vi "PathVelocityProfile.vi"(0 "Pose":dbl[](array[numeric]), 1 "time":dbl, 3 "intervalo":dbl=0.016, 5 "estimatives":T2, 9 "Path  Smooth":dbl[][](array[numeric]), 11 "V_max":dbl format="%#_13g", 13 "Accel":dbl=10.0, 14 "DesAccel":dbl=15.0) -> (4 "Time X":dbl[](array[numeric]), 6 "Velocities X":dbl[](array[numeric]), 8 "Time Y":dbl[](array[numeric]), 10 "Velocities Y":dbl[](array[numeric]))   [LabVIEW 2017]
uses:
  Controle/VelocityProfileState.ctl
  <vilib>/Analysis/_algsub.llb/Real Vector Norm.vi
  <vilib>/Analysis/coordinate.llb/Wrap Angle (scalar).vi
  <vilib>/Analysis/NI_AAL_Angle.lvlib
  <vilib>/Analysis/NI_AALPro.lvlib
panel:
  in  "est_vy":dbl
  in  "est_vx":dbl
  out "VelocityProfile Y":T1[](array[typedef])
  out "VelocityProfile X":T1[](array[typedef])
  out "Velocity Profile Y":cluster{dbl[], dbl[]}[](graph)
  out "Velocity Profile X":cluster{dbl[], dbl[]}[](graph)
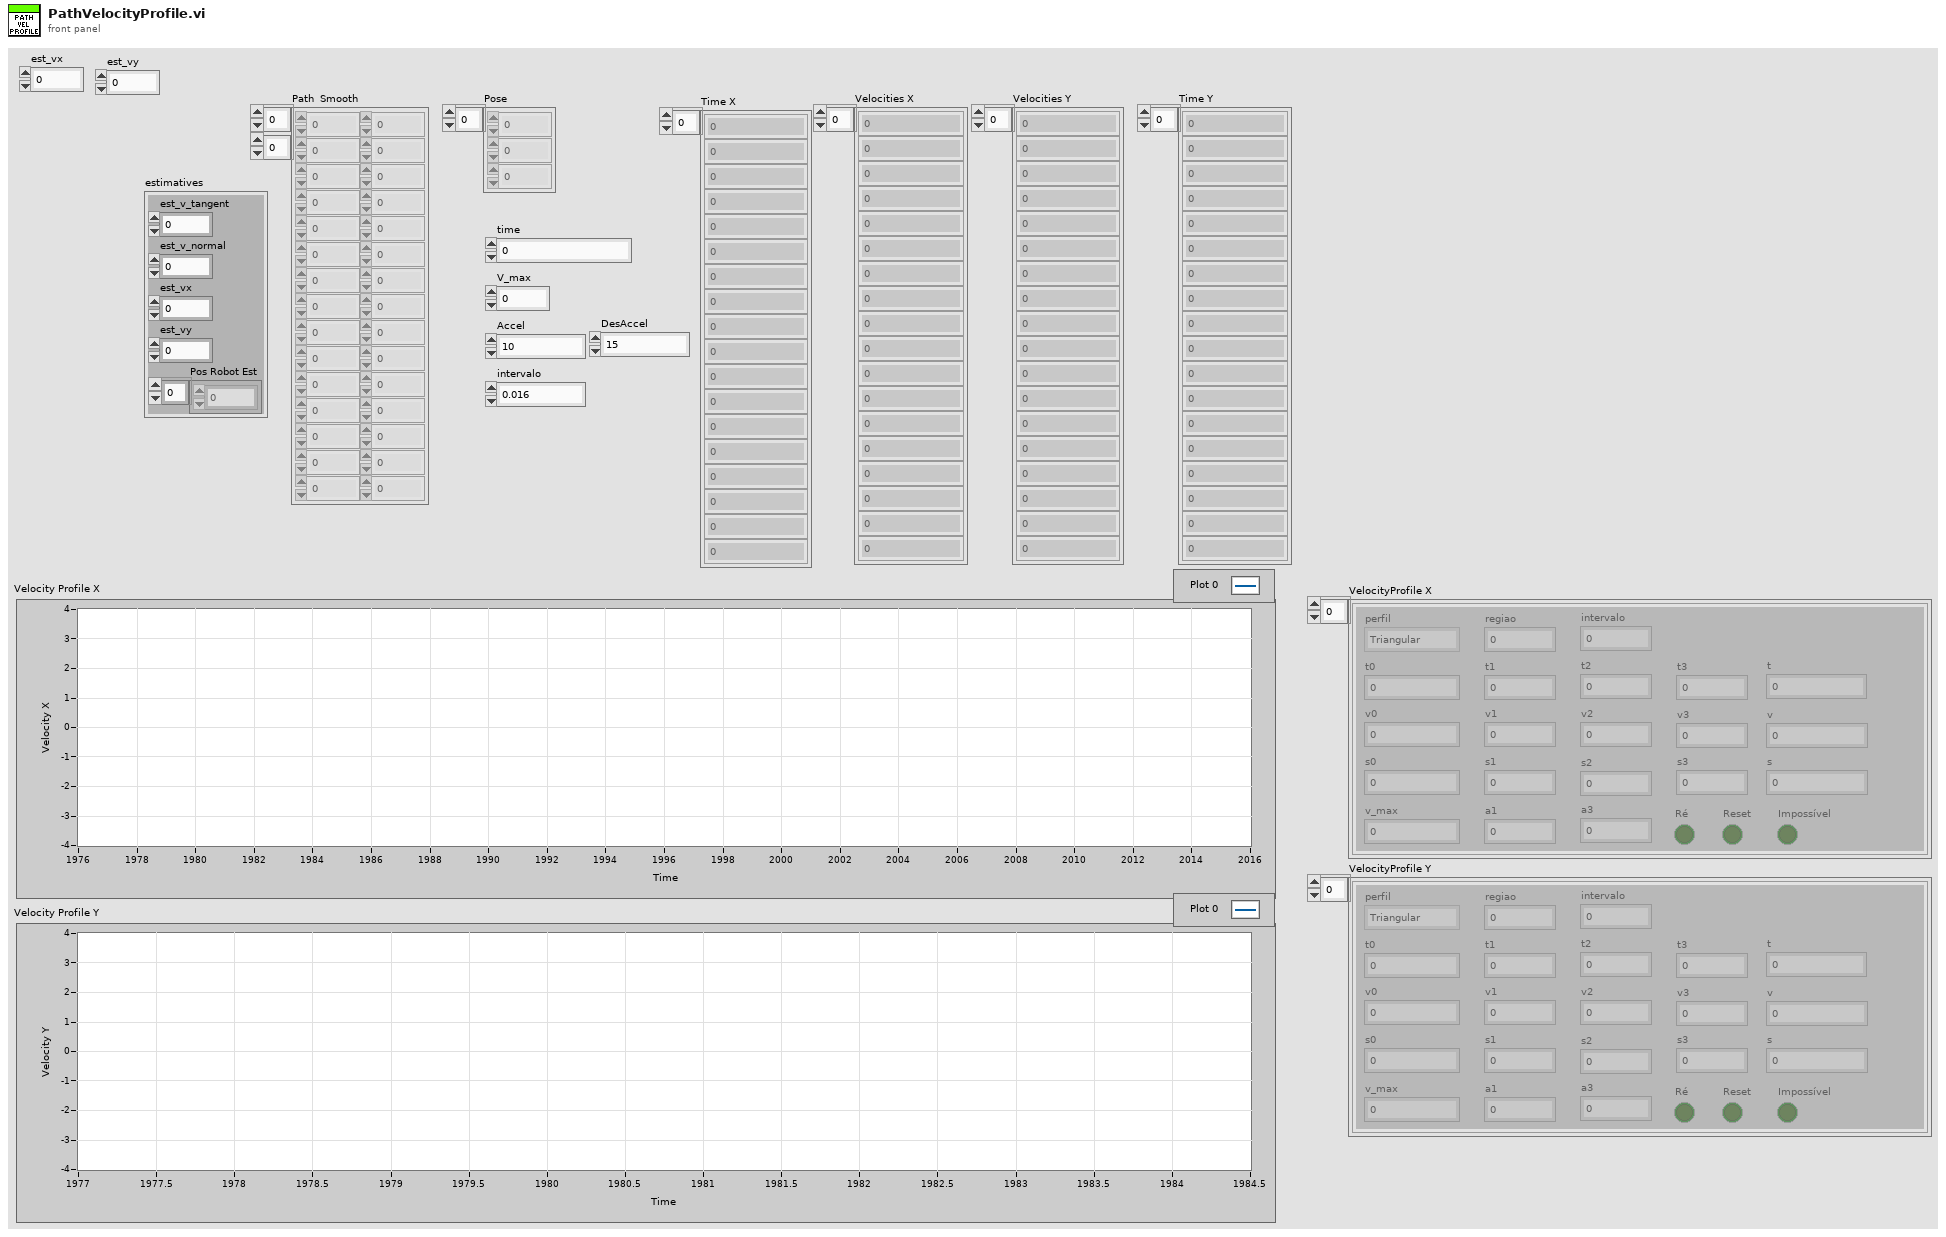
[diagram p1: front panel]
types:
  T1 = typedef "VelocityProfileState.ctl" = cluster{"t0":dbl, "t1":dbl, "t2":dbl, "t3":dbl, "v0":dbl, "v_max":dbl, "v3":dbl, "v2":dbl, "v1":dbl, "perfil":enum16{"Triangular", "Trapezoidal"}, "regiao":i32, "s0":dbl, "s1":dbl, "s2":dbl, "v":dbl, "t":dbl, "a1":dbl, "s3":dbl, "Reset":bool, "s":dbl, "a3":dbl, "Ré":bool, "Impossível":bool, "intervalo":dbl}
  T2 = cluster{"est_v_tangent":dbl, "est_v_normal":dbl, "est_vx":dbl, "est_vy":dbl, "Pos Robot Est":dbl[]}
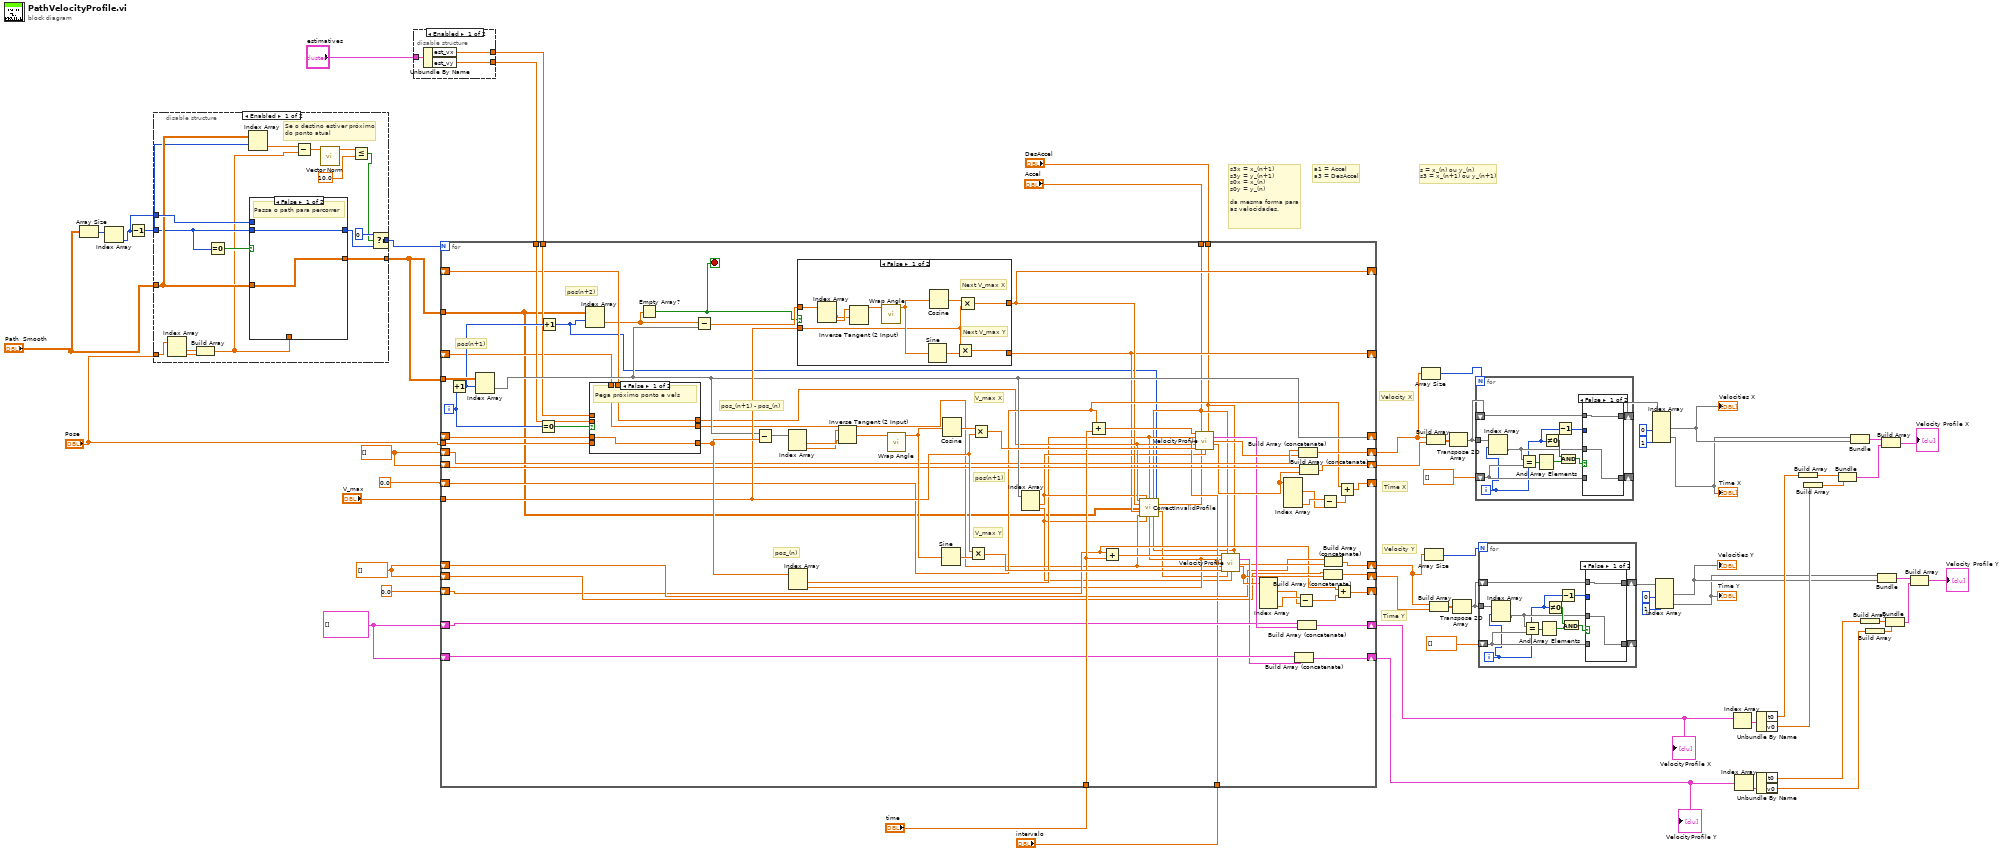
[diagram p0: block diagram]
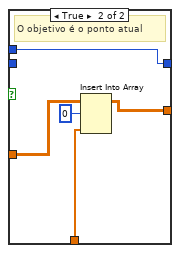
[diagram p2: hidden frame]
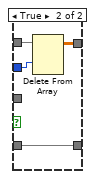
[diagram p4: hidden frame]
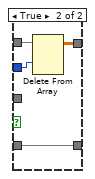
[diagram p5: hidden frame]
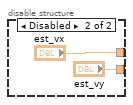
[diagram p6: hidden frame]
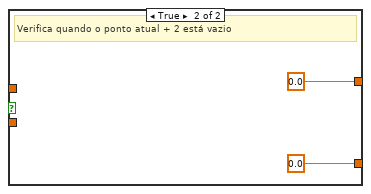
[diagram p7: hidden frame]
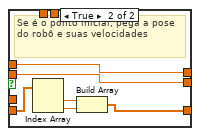
[diagram p8: hidden frame]
diagram:
  w48 = T1[] []
  w50 = dbl[] []
  w49 = dbl[] []
  # "s = x_(n) ou y_(n)\ns3 = x_(n+1) ou y_(n+1)"
  # "a1 = Accel\na3 = DesAccel"
  # "s3x = x_(n+1)\ns3y = y_(n+1)\ns0x = x_(n)\ns0y = y_(n)\n\nda mesma forma para\nas velocidades."
  # "Time X"
  # "Time Y"
  # "Velocity Y"
  # "Velocity X"
  n1 = Array Size(array="Path  Smooth") -> (size(s)=w53:i32[])
  n2 = Index Array(array=w53) -> (element=w6:i32)  [unwired: 1 in]
  n3 = Decrement(x=w6) -> (x-1=w3:i32)
  n4 = disable-structure shown="Enabled" {
    disable-tunnel: [w77 w85] -> w2
    disable-tunnel: w6 -> [w75 _]
    disable-tunnel: "Pose" -> [w74 _]
    disable-tunnel: [w71 w86] -> w1
    disable-tunnel: "Path  Smooth" -> [w68 w85]
    disable-tunnel: w3 -> [w67 w86]
    frame Enabled {
      # "Se o destino estiver próximo\ndo ponto atual"
      n5 = Index Array(array=w74) -> (element #1=w73:dbl, element #2=w72:dbl)  [unwired: 2 in]
      n6 = Build Array(w73, w72) -> (w65:dbl[])
      n7 = Equal To 0?(x=w67) -> (x = 0?=w76:bool)
      n8 = Index Array(array=w68, index (row)=w67) -> (element=w66:dbl[])  [unwired: 1 in]
      n9 = case shown="False" w76 {
        tunnel: [w78 w80] -> w77
        tunnel: w68 -> [w78 w82]
        tunnel: [w79 w84] -> w70
        tunnel: w67 -> [w79 _]
        tunnel: w75 -> [_ w84]
        tunnel: w65 -> [_ w83]
        frame False {
          # "Passa o path para percorrer"
        }
        frame True {
          # "O objetivo é o ponto atual"
          n10 = Insert Into Array(array=w82, index (row)=0, new element=w83) -> (w80:dbl[][])  [unwired: 1 in]
        }
      }
      n11 = Subtract(x=w66, y=w65) -> (x-y=w64:dbl[])
      n12 = call-poly <vilib>:"Vector Norm.vi"("Input Vector"=w64) -> ("norm"=w63:dbl)  [unwired: 9 in, 1 out]
      n13 = Less Or Equal?(x=w63, y=10.0) -> (x <= y?=w61:bool)
      n14 = Select(t=0, s=w61, f=w70) -> (s? t:f=w71:i32)
    }
    frame Disabled {
    }
  }
  n15 = disable-structure shown="Enabled" {
    disable-tunnel: "estimatives" -> [w89 _]
    disable-tunnel: [w88 "est_vx"] -> w52
    disable-tunnel: [w87 "est_vy"] -> w51
    frame Enabled {
      n16 = Unbundle By Name(w89) -> ("est_vx"=w88:dbl, "est_vy"=w87:dbl)
    }
    frame Disabled {
    }
  }
  n17 = for {
    N: w1 -> [_]
    tunnel: w2 -> [w143]
    tunnel: "Pose" -> [w161]
    shift-right: [w144] -> _
    shift-left: _ -> [w160]
    tunnel: "V_max" -> [w148]
    tunnel: "Accel" -> [w97]
    tunnel: "DesAccel" -> [w96]
    tunnel: w2 -> [w93]
    shift-right: [w112] -> _
    shift-left: 0.0 ("t3") -> [w114]
    shift-right: [w110] -> _
    shift-left: 0.0 ("t3") -> [w109]
    tunnel: "time" -> [w146]
    shift-right: [w137] -> w27
    shift-left: w49 -> [w142]
    shift-right: [w140] -> w30
    shift-left: w49 -> [w141]
    shift-right: [w118] -> w9
    shift-left: w50 -> [w116]
    shift-right: [w117] -> w10
    shift-left: w50 -> [w115]
    tunnel: w52 -> [w134]
    tunnel: w51 -> [w133]
    shift-right: [w106] -> _
    shift-left: _ -> [w132]
    shift-right: [w100] -> _
    shift-left: _ -> [w131]
    shift-right: [w123] -> w46
    shift-left: w48 -> [w126]
    shift-right: [w122] -> w45
    shift-left: w48 -> [w125]
    tunnel: "intervalo" -> [w108]
    i -> [w94]
    stop <- w135 stop-if-true
    # "pos(n+2)"
    # "pos(n+1)"
    # "pos(n+1)"
    # "pos_(n)"
    # "pos_(n+1) - pos_(n)"
    # "V_max Y"
    # "V_max X"
    n18 = Increment(x=w94) -> (x+1=w139:i32)
    n19 = Index Array(array=w143, index (row)=w139) -> (element=w144:dbl[])  [unwired: 1 in]
    n20 = Equal To 0?(x=w94) -> (x = 0?=w162:bool)
    n21 = Increment(x=w139) -> (x+1=w92:i32)
    n22 = Index Array(array=w93, index (row)=w92) -> (element=w95:dbl[])  [unwired: 1 in]
    n23 = case shown="False" w162 {
      tunnel: w161 -> [_ w183]
      tunnel: [w177 w180] -> w152
      tunnel: w160 -> [w177 _]
      tunnel: w134 -> [_ w179]
      tunnel: w133 -> [_ w178]
      tunnel: [w175 w179] -> w107
      tunnel: [w176 w178] -> w102
      tunnel: w132 -> [w175 _]
      tunnel: w131 -> [w176 _]
      frame False {
        # "Pega próximo ponto e vels"
      }
      frame True {
        # "Se é o ponto inicial, pega a pose\ndo robô e suas velocidades"
        n24 = Index Array(array=w183) -> (element #1=w182:dbl, element #2=w181:dbl)  [unwired: 2 in]
        n25 = Build Array(w182, w181) -> (w180:dbl[])
      }
    }
    n26 = Empty Array?(array=w95) -> (empty?=w135:bool)
    n27 = Subtract(x=w95, y=w144) -> (x-y=w149:dbl[])
    n28 = Subtract(x=w144, y=w152) -> (x-y=w158:dbl[])
    n29 = Index Array(array=w158) -> (element #1=w159:dbl, element #2=w157:dbl)  [unwired: 2 in]
    n30 = Index Array(array=w152) -> (element #1=w104:dbl, element #2=w103:dbl)  [unwired: 2 in]
    n31 = case shown="False" w135 {
      tunnel: w149 -> [w167 _]
      tunnel: w148 -> [w165 _]
      tunnel: [w164 0.0] -> w106
      tunnel: [w163 0.0] -> w100
      frame False {
        # "Next V_max Y"
        # "Next V_max X"
        n32 = Index Array(array=w167) -> (element #1=w166:dbl, element #2=w168:dbl)  [unwired: 2 in]
        n33 = Inverse Tangent (2 Input)(1:w166, 2:w168) -> (0:w169:dbl)
        n34 = call-poly <vilib>:"Wrap Angle.vi"("angle in"=w169) -> ("angle out"=w170:dbl)  [unwired: 9 in, 1 out]
        n35 = Sine(x=w170) -> (sin(x)=w172:dbl)
        n36 = Cosine(x=w170) -> (cos(x)=w171:dbl)
        n37 = Multiply(x=w165, y=w172) -> (x*y=w163:dbl)
        n38 = Multiply(x=w171, y=w165) -> (x*y=w164:dbl)
      }
      frame True {
        # "Verifica quando o ponto atual + 2 está vazio"
      }
    }
    n39 = Inverse Tangent (2 Input)(1:w159, 2:w157) -> (0:w156:dbl)
    n40 = call-poly <vilib>:"Wrap Angle.vi"("angle in"=w156) -> ("angle out"=w155:dbl)  [unwired: 9 in, 1 out]
    n41 = Sine(x=w155) -> (sin(x)=w153:dbl)
    n42 = Cosine(x=w155) -> (cos(x)=w154:dbl)
    n43 = Multiply(x=w148, y=w153) -> (x*y=w150:dbl)
    n44 = Multiply(x=w154, y=w148) -> (x*y=w151:dbl)
    n45 = Index Array(array=w144) -> (element #1=w105:dbl, element #2=w101:dbl)  [unwired: 2 in]
    n46 = Add(x=w114, y=w146) -> (x+y=w147:dbl)
    n47 = Add(x=w109, y=w146) -> (x+y=w145:dbl)
    n48 = call "CorrectInvalidProfile.vi"("v0x"=w107, "s3x"=w105, "s0x"=w104, "a1"=w97, "index"=w92, "v3x"=w106, "Path  Smooth"=w93, "v3y"=w100, "v0y"=w102, "s3y"=w101, "s0y"=w103, "a3"=w96) -> ("New v3x"=w98:dbl, "New v3y"=w99:dbl)  [unwired: 2 in]
    n49 = call "VelocityProfile.vi"("t"=w147, "a1"=w97, "a3"=w96, "s"=w104, "intervalo"=w108, "v_est"=w107, "v_max"=w151, "v3"=w98, "s3"=w105) -> ("VelocityProfileState Out"=w127:T1, "Velocities"=w138:dbl[], "Time"=w136:dbl[])  [unwired: 3 in, 1 out]
    n50 = call "VelocityProfile.vi"("t"=w145, "a1"=w97, "a3"=w96, "s"=w103, "intervalo"=w108, "v_est"=w102, "v_max"=w150, "v3"=w99, "s3"=w101) -> ("VelocityProfileState Out"=w124:T1, "Velocities"=w121:dbl[], "Time"=w119:dbl[])  [unwired: 3 in, 1 out]
    n51 = Index Array(array=w119) -> (element #1=w129:dbl, element #4=w130:dbl)  [unwired: 4 in, 2 out]
    n52 = Index Array(array=w136) -> (element #1=w120:dbl, element #4=w128:dbl)  [unwired: 4 in, 2 out]
    n53 = Build Array (concatenate)(w125, w124) -> (w122:T1[])
    n54 = Subtract(x=w130, y=w129) -> (x-y=w111:dbl)
    n55 = Build Array (concatenate)(w126, w127) -> (w123:T1[])
    n56 = Build Array (concatenate)(w142, w138) -> (w137:dbl[])
    n57 = Build Array (concatenate)(w141, w136) -> (w140:dbl[])
    n58 = Subtract(x=w128, y=w120) -> (x-y=w113:dbl)
    n59 = Build Array (concatenate)(w115, w119) -> (w117:dbl[])
    n60 = Build Array (concatenate)(w116, w121) -> (w118:dbl[])
    n61 = Add(x=w109, y=w111) -> (x+y=w110:dbl)
    n62 = Add(x=w114, y=w113) -> (x+y=w112:dbl)
  }
  "VelocityProfile X" <- w46
  "VelocityProfile Y" <- w45
  n63 = Array Size(array=w27) -> (size(s)=w24:i32)
  n64 = Array Size(array=w9) -> (size(s)=w13:i32)
  n65 = Build Array(w27, w30) -> (w23:dbl[][])
  n66 = Build Array(w9, w10) -> (w14:dbl[][])
  n67 = Transpose 2D Array(2D array=w23) -> (transposed array=w22:dbl[][])
  n68 = Transpose 2D Array(2D array=w14) -> (transposed array=w15:dbl[][])
  n69 = for {
    N: w24 -> [_]
    tunnel: w22 -> [w187]
    shift-right: [w195] -> _
    shift-left: dbl[] [] -> [w194]
    shift-right: [w188] -> w25
    shift-left: w22 -> [w189]
    i -> [w184]
    n70 = Index Array(array=w187, index (row)=w184) -> (element=w186:dbl[])  [unwired: 1 in]
    n71 = Equal?(x=w186, y=w194) -> (x = y?=w193:bool[])
    n72 = And Array Elements(Boolean array=w193) -> (logical AND=w192:bool)
    n73 = Not Equal To 0?(x=w184) -> (x != 0?=w191:bool)
    n74 = Decrement(x=w184) -> (x-1=w185:i32)
    n75 = And(x=w191, y=w192) -> (x .and. y?=w190:bool)
    n76 = case shown="False" w190 {
      tunnel: w186 -> [w197 _]
      tunnel: [w197 w201] -> w195
      tunnel: w194 -> [_ w201]
      tunnel: w189 -> [w196 w200]
      tunnel: [w196 w199] -> w188
      tunnel: w185 -> [_ w198]
      frame False {
      }
      frame True {
        n77 = Delete From Array(array=w200, index (row)=w198) -> (array with subset deleted=w199:dbl[][])  [unwired: 2 in, 1 out]
      }
    }
  }
  n78 = for {
    N: w13 -> [_]
    tunnel: w15 -> [w205]
    shift-right: [w213] -> _
    shift-left: dbl[] [] -> [w212]
    shift-right: [w206] -> w12
    shift-left: w15 -> [w207]
    i -> [w202]
    n79 = Index Array(array=w205, index (row)=w202) -> (element=w204:dbl[])  [unwired: 1 in]
    n80 = Equal?(x=w204, y=w212) -> (x = y?=w211:bool[])
    n81 = And Array Elements(Boolean array=w211) -> (logical AND=w210:bool)
    n82 = Not Equal To 0?(x=w202) -> (x != 0?=w209:bool)
    n83 = Decrement(x=w202) -> (x-1=w203:i32)
    n84 = And(x=w209, y=w210) -> (x .and. y?=w208:bool)
    n85 = case shown="False" w208 {
      tunnel: w204 -> [w215 _]
      tunnel: [w215 w219] -> w213
      tunnel: w212 -> [_ w219]
      tunnel: w207 -> [w214 w218]
      tunnel: [w214 w217] -> w206
      tunnel: w203 -> [_ w216]
      frame False {
      }
      frame True {
        n86 = Delete From Array(array=w218, index (row)=w216) -> (array with subset deleted=w217:dbl[][])  [unwired: 2 in, 1 out]
      }
    }
  }
  n87 = Index Array(array=w25, index (col) #1=0 ("disabled index (col)"), index (col) #2=1 ("index (col)")) -> (element #1=w29:dbl[], element #2=w28:dbl[])  [unwired: 2 in]
  "Velocities X" <- w29
  "Time X" <- w28
  n88 = Index Array(array=w12, index (col) #1=0 ("disabled index (col)"), index (col) #2=1 ("index (col)")) -> (element #1=w8:dbl[], element #2=w7:dbl[])  [unwired: 2 in]
  "Velocities Y" <- w8
  "Time Y" <- w7
  n89 = Index Array(array=w46) -> (element=w44:T1)  [unwired: 1 in]
  n90 = Index Array(array=w45) -> (element=w43:T1)  [unwired: 1 in]
  n91 = Unbundle By Name(w44) -> ("t0"=w36:dbl, "v0"=w35:dbl)
  n92 = Unbundle By Name(w43) -> ("t0"=w32:dbl, "v0"=w31:dbl)
  n93 = Build Array(w36) -> (w37:dbl[])
  n94 = Build Array(w35) -> (w38:dbl[])
  n95 = Bundle(w37, w38) -> (w18:cluster{dbl[], dbl[]})  [unwired: 1 in]
  n96 = Bundle(w28, w29) -> (w42:cluster{dbl[], dbl[]})  [unwired: 1 in]
  n97 = Build Array(w32) -> (w33:dbl[])
  n98 = Build Array(w31) -> (w34:dbl[])
  n99 = Bundle(w7, w8) -> (w40:cluster{dbl[], dbl[]})  [unwired: 1 in]
  n100 = Build Array(w42, w18) -> (→"Velocity Profile X":cluster{dbl[], dbl[]}[])
  n101 = Bundle(w33, w34) -> (w19:cluster{dbl[], dbl[]})  [unwired: 1 in]
  n102 = Build Array(w40, w19) -> (→"Velocity Profile Y":cluster{dbl[], dbl[]}[])
